vi "ti2_err2msg.vi"(11 "Error Code":i32) -> (3 "Error Message":string)   [LabVIEW 2023, in "ti2lv.lvlib"]
uses:
  ti2lv.lvlib
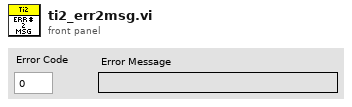
[diagram p1: front panel]
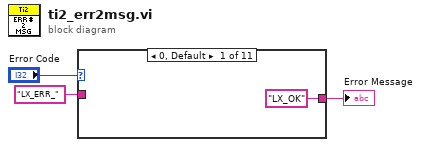
[diagram p0: block diagram]
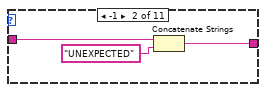
[diagram p2: hidden frame]
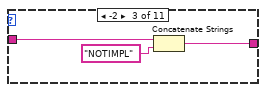
[diagram p3: hidden frame]
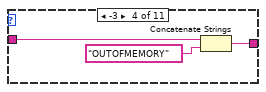
[diagram p4: hidden frame]
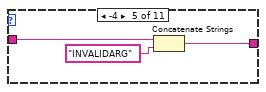
[diagram p5: hidden frame]
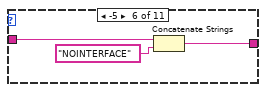
[diagram p6: hidden frame]
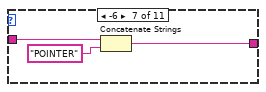
[diagram p7: hidden frame]
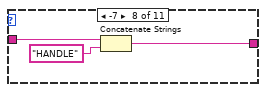
[diagram p8: hidden frame]
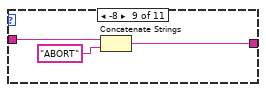
[diagram p9: hidden frame]
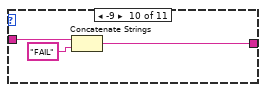
[diagram p10: hidden frame]
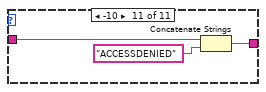
[diagram p11: hidden frame]
diagram:
  n1 = case shown="0, Default" "Error Code" {
    tunnel: ["LX_OK" ("Error Message") w5 w8 w11 w14 w17 w20 w23 w26 w29 w32] -> w2
    tunnel: "LX_ERR_" ("Error Message") -> [_ w7 w10 w13 w16 w19 w22 w25 w28 w31 w34]
    frame 0, Default {
    }
    frame -1 {
      n2 = Concatenate Strings(w7, "UNEXPECTED" ("string")) -> (w5:string)
    }
    frame -2 {
      n3 = Concatenate Strings(w10, "NOTIMPL" ("string")) -> (w8:string)
    }
    frame -3 {
      n4 = Concatenate Strings(w13, "OUTOFMEMORY" ("string")) -> (w11:string)
    }
    frame -4 {
      n5 = Concatenate Strings(w16, "INVALIDARG" ("string")) -> (w14:string)
    }
    frame -5 {
      n6 = Concatenate Strings(w19, "NOINTERFACE" ("string")) -> (w17:string)
    }
    frame -6 {
      n7 = Concatenate Strings(w22, "POINTER" ("string")) -> (w20:string)
    }
    frame -7 {
      n8 = Concatenate Strings(w25, "HANDLE" ("string")) -> (w23:string)
    }
    frame -8 {
      n9 = Concatenate Strings(w28, "ABORT" ("string")) -> (w26:string)
    }
    frame -9 {
      n10 = Concatenate Strings(w31, "FAIL" ("string")) -> (w29:string)
    }
    frame -10 {
      n11 = Concatenate Strings(w34, "ACCESSDENIED" ("string")) -> (w32:string)
    }
  }
  "Error Message" <- w2
